vi "Configure Modulation (FM).vi"(0 "VISA resource name":refnum<visa-resource-name>, 1 "Enable FM (T: Enable)":bool=TRUE, 2 "Modulation Waveform (0: Sine)":u16(ring) items=["Sine", "Square", "Ramp", "Noise", "User Waveform", "Edit Memory", "EFile"], 5 "Channel (1: Channel 1)":u16(ring)=1 items=["Channel 1"=1, "Channel 2"=2], 7 "FM Source (0: Internal)":u16(ring) items=["Internal", "External"], 9 "Peak Deviation (100.00 Hz)":dbl=100.0, 11 "error in (no error)":errorcluster, 12 "Modulation Frequency (100.00 Hz)":dbl=100.0, 13 "User Waveform (0)":i32, 14 "EFile Name (\"\")":string) -> (4 "VISA resource name out":refnum<visa-resource-name>, 15 "error out":errorcluster)   [LabVIEW 2016, in "Tektronix AFG 1000 Series.lvlib"]
doc: "Configures and enables frequency modulation (FM). In FM, the frequency of the carrier is varied by the frequency of the modulating waveform."
uses:
  Tektronix AFG 1000 Series.lvlib
panel:
  # "Internal FM Settings"
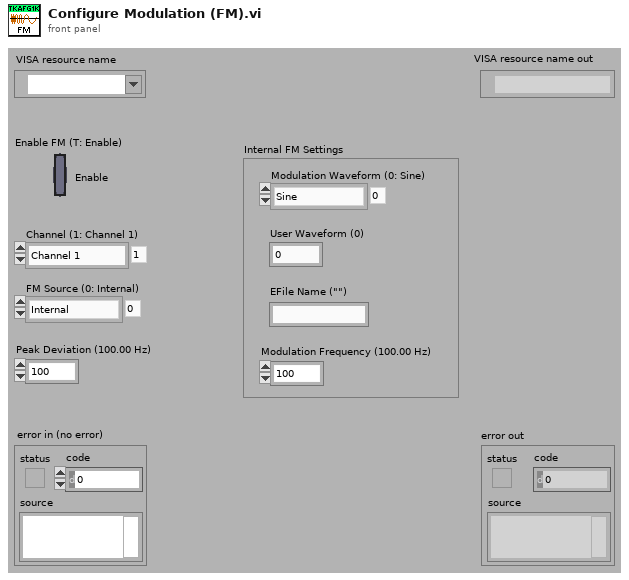
[diagram p1: front panel]
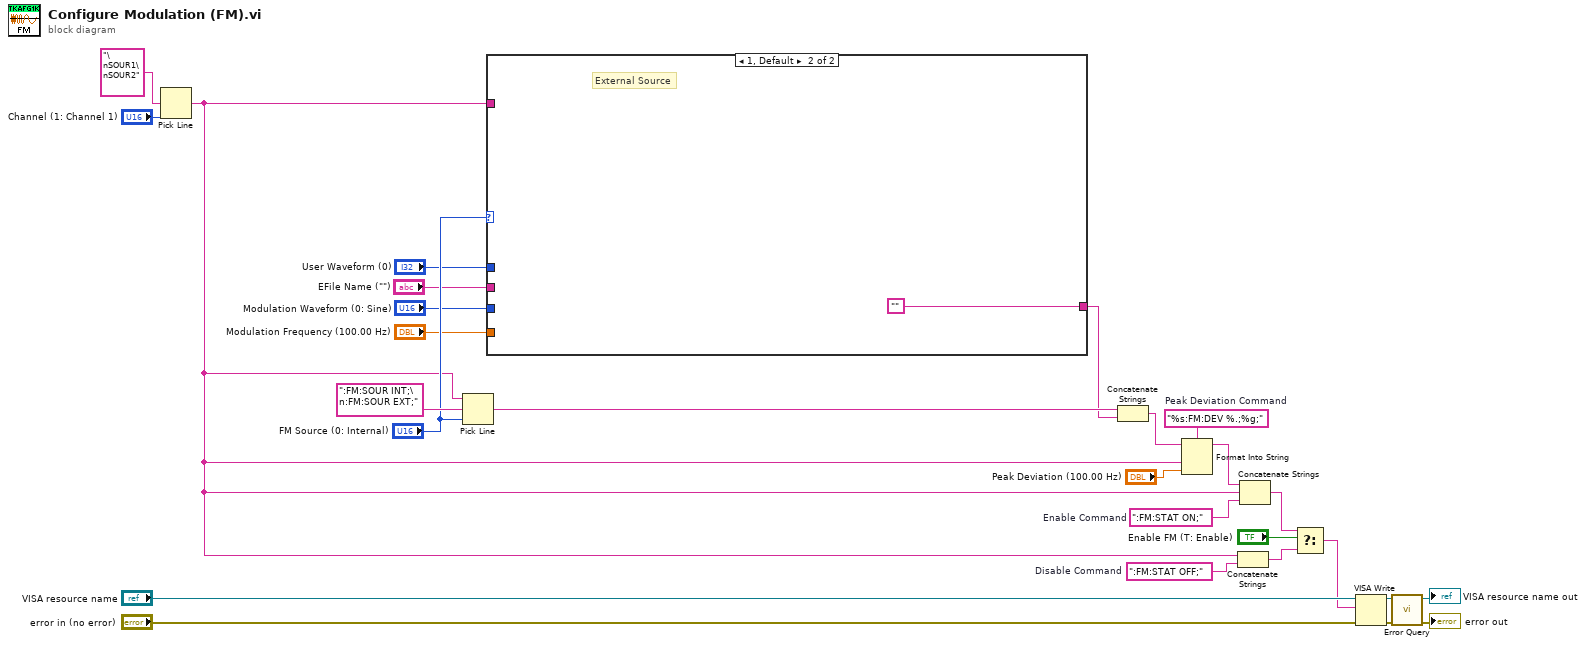
[diagram p0: block diagram]
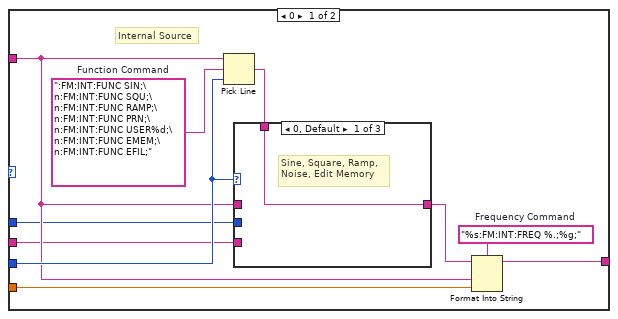
[diagram p2: hidden frame]
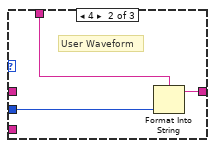
[diagram p3: hidden frame]
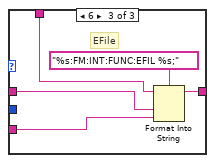
[diagram p4: hidden frame]
diagram:
  w18 = ":FM:STAT ON;"  # Enable Command
  w21 = "%s:FM:DEV %.;%g;"  # Peak Deviation Command
  w15 = ":FM:STAT OFF;"  # Disable Command
  n1 = Pick Line(multi-line string="\nSOUR1\nSOUR2" ("string (\"\")"), line index="Channel (1: Channel 1)") -> (output string=w2:string)  [unwired: 1 in]
  n2 = Pick Line(string ("")=w2, multi-line string=":FM:SOUR INT;\n:FM:SOUR EXT;" ("Source Command"), line index="FM Source (0: Internal)") -> (output string=w9:string)
  n3 = case shown="1, Default" "FM Source (0: Internal)" {
    tunnel: w2 -> [w30 _]
    tunnel: [w35 ""] -> w3
    tunnel: "Modulation Waveform (0: Sine)" -> [w31 _]
    tunnel: "Modulation Frequency (100.00 Hz)" -> [w34 _]
    tunnel: "User Waveform (0)" -> [w29 _]
    tunnel: "EFile Name (\"\")" -> [w28 _]
    frame 0 {
      w36 = "%s:FM:INT:FREQ %.;%g;"  # Frequency Command
      w37 = ":FM:INT:FUNC SIN;\n:FM:INT:FUNC SQU;\n:FM:INT:FUNC RAMP;\n:FM:INT:FUNC PRN;\n:FM:INT:FUNC USER%d;\n:FM:INT:FUNC EMEM;\n:FM:INT:FUNC EFIL;"  # Function Command
      # "Internal Source"
      n4 = Pick Line(string ("")=w30, multi-line string=w37, line index=w31) -> (output string=w33:string)
      n5 = case shown="0, Default" w31 {
        tunnel: w33 -> [w38 w41 w45]
        tunnel: [w38 w40 w46] -> w32
        tunnel: w30 -> [_ _ w43]
        tunnel: w29 -> [_ w39 _]
        tunnel: w28 -> [_ _ w42]
        frame 0, Default {
          # "Sine, Square, Ramp,\nNoise, Edit Memory"
        }
        frame 4 {
          # "User Waveform"
          n6 = Format Into String(format string=w41, w39) -> (resulting string=w40:string)  [unwired: 2 in, 1 out]
        }
        frame 6 {
          # "EFile"
          n7 = Format Into String(format string="%s:FM:INT:FUNC:EFIL %s;", initial string=w45, w43, w42) -> (resulting string=w46:string)  [unwired: 1 in, 1 out]
        }
      }
      n8 = Format Into String(format string=w36, initial string=w32, w30, w34) -> (resulting string=w35:string)  [unwired: 1 in, 1 out]
    }
    frame 1, Default {
      # "External Source"
    }
  }
  n9 = Concatenate Strings(w9, w3) -> (w8:string)
  n10 = Format Into String(format string=w21, initial string=w8, w2, "Peak Deviation (100.00 Hz)") -> (resulting string=w19:string)  [unwired: 1 in, 1 out]
  n11 = Concatenate Strings(w2, w15) -> (w13:string)
  n12 = Concatenate Strings(w19, w2, w18) -> (w11:string)
  n13 = Select(t=w11, s="Enable FM (T: Enable)", f=w13) -> (s? t:f=w12:string)
  n14 = VISA Write(VISA resource name="VISA resource name", write buffer=w12, error in (no error)="error in (no error)") -> (VISA resource name out=w24:refnum<visa-resource-name>, error out=w25:errorcluster)  [unwired: 1 out]
  n15 = call "Error Query.vi"("error in (no error)"=w25, "VISA resource name"=w24) -> ("error out"=→"error out":errorcluster, "VISA resource name out"=→"VISA resource name out":refnum<visa-resource-name>)  [unwired: 6 in, 2 out]
